vi "Implementation Error.vi"(8 "error in (no error)":errorcluster) -> (0 "error out":errorcluster)   [LabVIEW 2019, in "Abstract Spectrometer.lvclass"]
uses:
  Abstract Spectrometer.lvclass
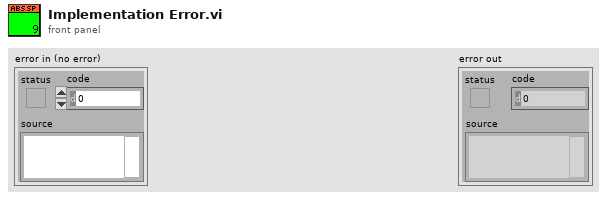
[diagram p1: front panel]
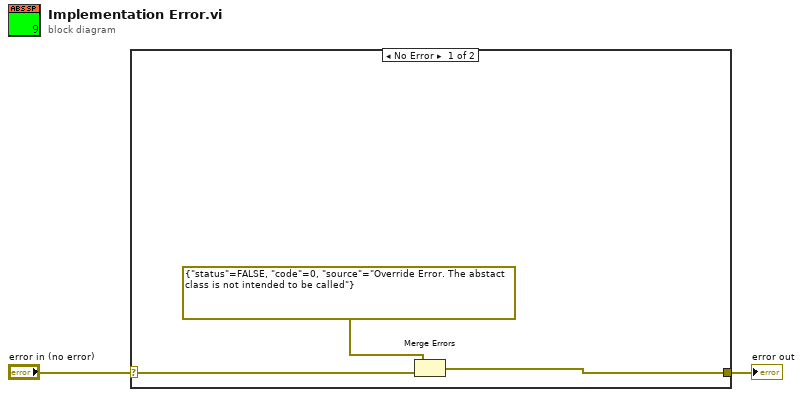
[diagram p0: block diagram]
diagram:
  n1 = case shown="No Error" "error in (no error)" {
    selector: "error in (no error)" -> [w5 w6]
    tunnel: [w4 w6] -> w1
    frame No Error {
      n2 = Merge Errors(errorcluster {"status"=FALSE, "code"=0, "source"="Override Error. The abstact class is not intended to be called"} ("error in"), w5) -> (w4:errorcluster)
    }
    frame Error {
    }
  }
  "error out" <- w1
